vi "altwaitall.vi"(8 "error in (no error)":errorcluster, 9 "Theta enabled":bool, 11 "VISA Refnum in":refnum<visa-resource-name>) -> (0 "error out":errorcluster, 3 "VISA Refnum out":refnum<visa-resource-name>)   [LabVIEW 2020]
uses:
  haltnow.vi
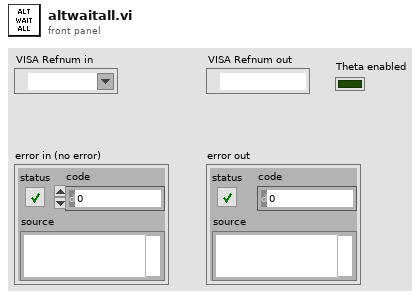
[diagram p1: front panel]
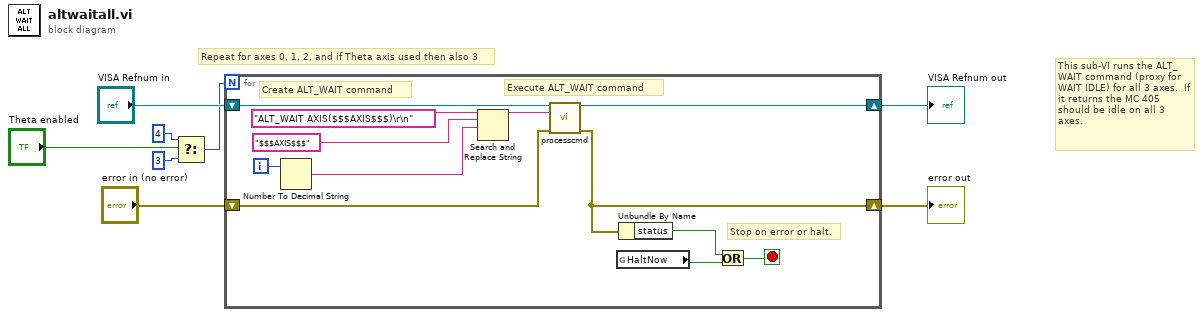
[diagram p0: block diagram]
diagram:
  # "This sub-VI runs the ALT_WAIT command (proxy for WAIT IDLE) for all 3 axes.  If it returns the MC 405 should be idle on all 3 axes."
  # "Repeat for axes 0, 1, 2, and if Theta axis used then also 3"
  n1 = Select(t=4, s="Theta enabled", f=3) -> (s? t:f=w1:i32)
  n2 = for {
    N: w1 -> [_]
    shift-right: [w14] -> w6
    shift-left: "VISA Refnum in" -> [w15]
    shift-right: [w12] -> w8
    shift-left: "error in (no error)" -> [w13]
    i -> [w20]
    stop <- w9 stop-if-true
    # "Stop on error or halt."
    # "Execute ALT_WAIT command"
    # "Create ALT_WAIT command"
    n3 = Number To Decimal String(number=w20) -> (decimal integer string=w19:string)  [unwired: 1 in]
    n4 = Search and Replace String(input string="ALT_WAIT AXIS($$$AXIS$$$)\r\n" ("write buffer"), search string="$$$AXIS$$$", replace string=w19) -> (result string=w16:string)  [unwired: 5 in, 3 out]
    n5 = call "processcmd.vi"("VISA Refnum in"=w15, "write buffer"=w16, "error in (no error)"=w13) -> ("VISA Refnum out"=w14:refnum<visa-resource-name>, "error out"=w12:errorcluster)  [unwired: 10 in, 1 out]
    n6 = global read "haltnow.vi" "HaltNow"() -> (w10:bool)
    n7 = Unbundle By Name(w12) -> ("status"=w11:bool)
    n8 = Or(x=w11, y=w10) -> (x .or. y?=w9:bool)
  }
  "error out" <- w8
  "VISA Refnum out" <- w6
